vi "subSound.vi"(0 "Array 2":path[](array[path]), 1 "Array":bool[](array[boolean])) -> ()   [LabVIEW 2021]
doc: "This VI illustrates how to play a sound file directly to the speakers. It uses Play Sound File.vi which opens a file and starts playing immediately and asynchronously (as opposed to the method shown in Sound File to Sound Output.vi example)."
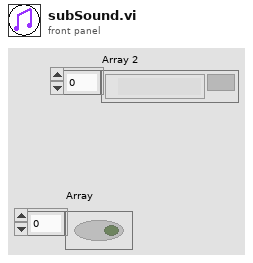
[diagram p1: front panel]
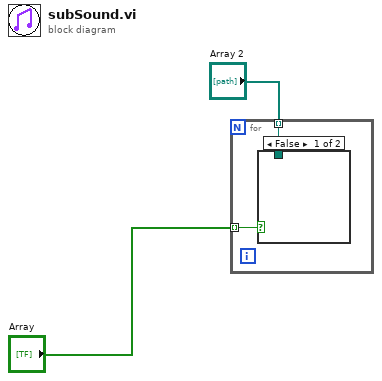
[diagram p0: block diagram]
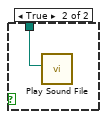
[diagram p2: hidden frame]
diagram:
  n1 = for {
    tunnel: "Array 2" -> [w4] mode=indexing
    tunnel: "Array" -> [w3] mode=indexing
    n2 = case shown="False" w3 {
      tunnel: w4 -> [_ w5]
      frame False {
      }
      frame True {
        n3 = call <vilib>:"Play Sound File.vi"("path"=w5) -> ()  [unwired: 9 in, 2 out]
      }
    }
  }
